vi "ecg_ncs_v1d.vi"() -> ()   [LabVIEW 2016]
uses:
  <instrlib>/niUSRP/niUSRP Timestamp.ctl
  C:/Program Files/National Instruments/LabVIEW 2016/examples/Instrument IO/Serial/support/Serial - Settings.ctl
  <vilib>/Analysis/coordinate.llb/Wrap Angle (array).vi
  <instrlib>/niUSRP/niUSRP Configure Time Start Trigger.vi
  <vilib>/Analysis/3filter.llb/Butterworth Filter (DBL).vi
  <vilib>/Instr/_visa.llb/VISA Configure Serial Port (Instr).vi
  <instrlib>/niUSRP/niUSRP Write Tx Data (2D CDB).vi
  <instrlib>/niUSRP/niUSRP Fetch Rx Data (2D CDB).vi
  <vilib>/measure/NI_MABase.lvlib
  <vilib>/Analysis/NI_AALBase.lvlib
  <vilib>/Analysis/NI_AALPro.lvlib
  <vilib>/Analysis/NI_AAL_Angle.lvlib
panel:
  out "size(s) 5":i32=800
  in  "Stop":bool
  out "size(s) 4":i32=800
  out "x/y":dbl=2000.0
  out "size(s) 3":i32=20000
  out "size(s) 2":i32=10
  out "Poor Sensor Quality: \nSensor off":bool=TRUE
  out "Poor Sensor Quality: \nSensor on":bool
  out "Heart Rate 2":u16[](array[numeric])=[71]
  out "Stop Loop":bool
  out "Loop index":i32=135
  out "size(s)":i32=384
  in  "Read Count":u32=800
  out "return count":u32=800
  out "Serial Settings:Number of Bytes at Serial Port":u32=8
  in  "Serial Settings":T1={"baud rate"=57600, "data bits"=8, "parity"=enum."None", "stop bits"=10, "flow control"=0} {"flow control" items=["None"=0, "XON/XOFF"=1, "RTS/CTS"=2, "DTR/DSR"=4]; "stop bits" items=["1.0"=10, "1.5"=15, "2.0"=20]; "data bits" min=5 max=8 step=1; "baud rate" items=["75"=75, "110"=110, "134"=134, "150"=150, "300"=300, "600"=600, "1200"=1200, "1800"=1800, "2400"=2400, "4800"=4800, "7200"=7200, "9600"=9600, "14400"=14400, "19200"=19200, "28800"=28800, "38400"=38400, "56000"=56000, "57600"=57600, "115200"=115200, "128000"=128000, "230400"=230400]}
  in  "VISA resource name":refnum<visa-resource-name>="bmd101"
  in  "?":enum32{"ECG", "Heart Rate"}(tab)
  out "?":i16(graph)=77
  out "?":u8[](graph)=[71]
  in  "File Name":string="Test"
  in  "order1":i32=5
  in  "Path":path=path "D:/Research/SummerFall17Spring18/CnC/NCS/EcgNcsCorrelation"
  in  "Low-Pass Freq":dbl=200.0 format="%#_13g"
  in  "Sampling Rate":i32=500
  out "Gain":dbl=-15.0
  out "Bandwidth":dbl=56000000.0
  out "Coerced Carrier Frequency":dbl=2000000000.0 format="%#.17g"
  out "Coerced Tx IQ rate":dbl=1000000.0
  out "Coerced Rx IQ rate":dbl=1000000.0
  out "error IO":errorcluster={"status"=FALSE, "code"=-1074118647, "source"=""}
  in  "Rx Number of Samples":i32=20000
  in  "Tab Control 2":enum32{"NI-294x/295x", "NI-2900/2901"}(tab)=enum."NI-2900/2901"
  in  "channel 0 carrier\n frequency [Hz]":dbl=2000000000.0 format="%#_6p"
  in  "Rx carrier frequency [Hz]":dbl=2000000000.0 format="%#_6p"
  in  "Tx carrier frequency [Hz]":dbl=1000000000.0 format="%#_6p"
  in  "Start Trigger Time":T2={"whole seconds"=1, "fractional seconds"=0.0}
  out "Tx Active Antenna":string="TX1"
  in  "Tab Control":T3(tab)
  out "NCS tag Amp":dbl[](graph)=[0.011680657018198379]
  out "NCS tag Phase":dbl[](graph)=[-1.312166394909216]
  out "Tag Amp":dbl[](graph)
  out "Tag Phase":dbl[](graph)
  out "Tx Waveform Graph":waveform(dbl)[](graph)
  in  "Channel 0\nTone Amplitude":dbl=0.707 step=0.05 format="%#.6g"
  in  "Channel 0 \nTone Frequency":dbl=5000.0 format="%#_6p"
  in  "Waveform Size":dbl=20000.0
  in  "Rx Active Antenna":string="RX2"
  in  "Device Name":refnum<k15>="MyB200"
  in  "Tx Gain":dbl=28.0 format="%#_6f"
  in  "Tx IQ Rate":dbl=1000000.0 format="%#_6p"
  in  "Rx Gain":dbl=32.0 format="%#_6f"
  in  "Rx IQ Rate":dbl=1000000.0 format="%#_6p"
  # "Rx Settings"
  # "Tx Settings"
  # "Note that on the NI-2900 and NI-2901, both Rx channels share an LO and both Tx channels share an LO. However, on the NI-294x/295x devices, Rx and Tx of channel 0 share an LO and Rx and Tx of channel 1 share an LO."
  # "This Tx graph should always have end and start tied up since this is being sent in a loop continuously. Otherwise phase jumps will be noticed."
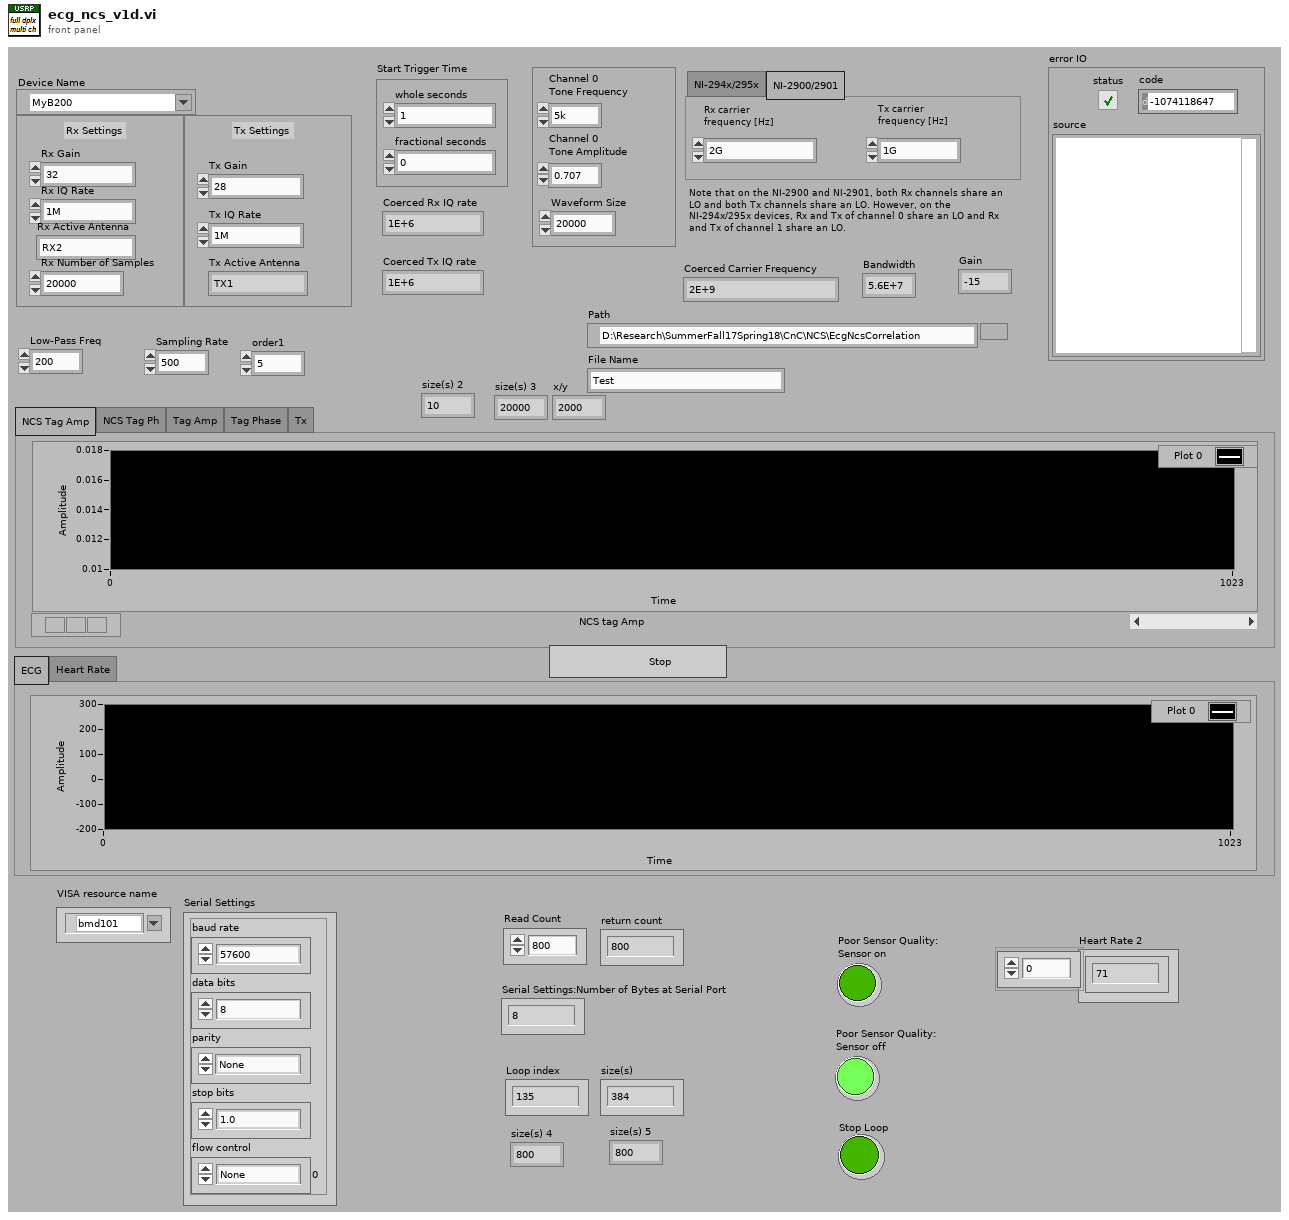
[diagram p1: front panel]
types:
  T1 = typedef "Serial - Settings.ctl" = cluster{"baud rate":u32, "data bits":u16, "parity":enum16{"None", "Odd", "Even", "Mark", "Space"}, "stop bits":u16, "flow control":u16}
  T2 = typedef "niUSRP Timestamp.ctl" = cluster{"whole seconds":u64, "fractional seconds":dbl}
  T3 = enum32{"NCS Tag Amp", "NCS Tag Ph", "Tag Amp", "Tag Phase", "Tx"}
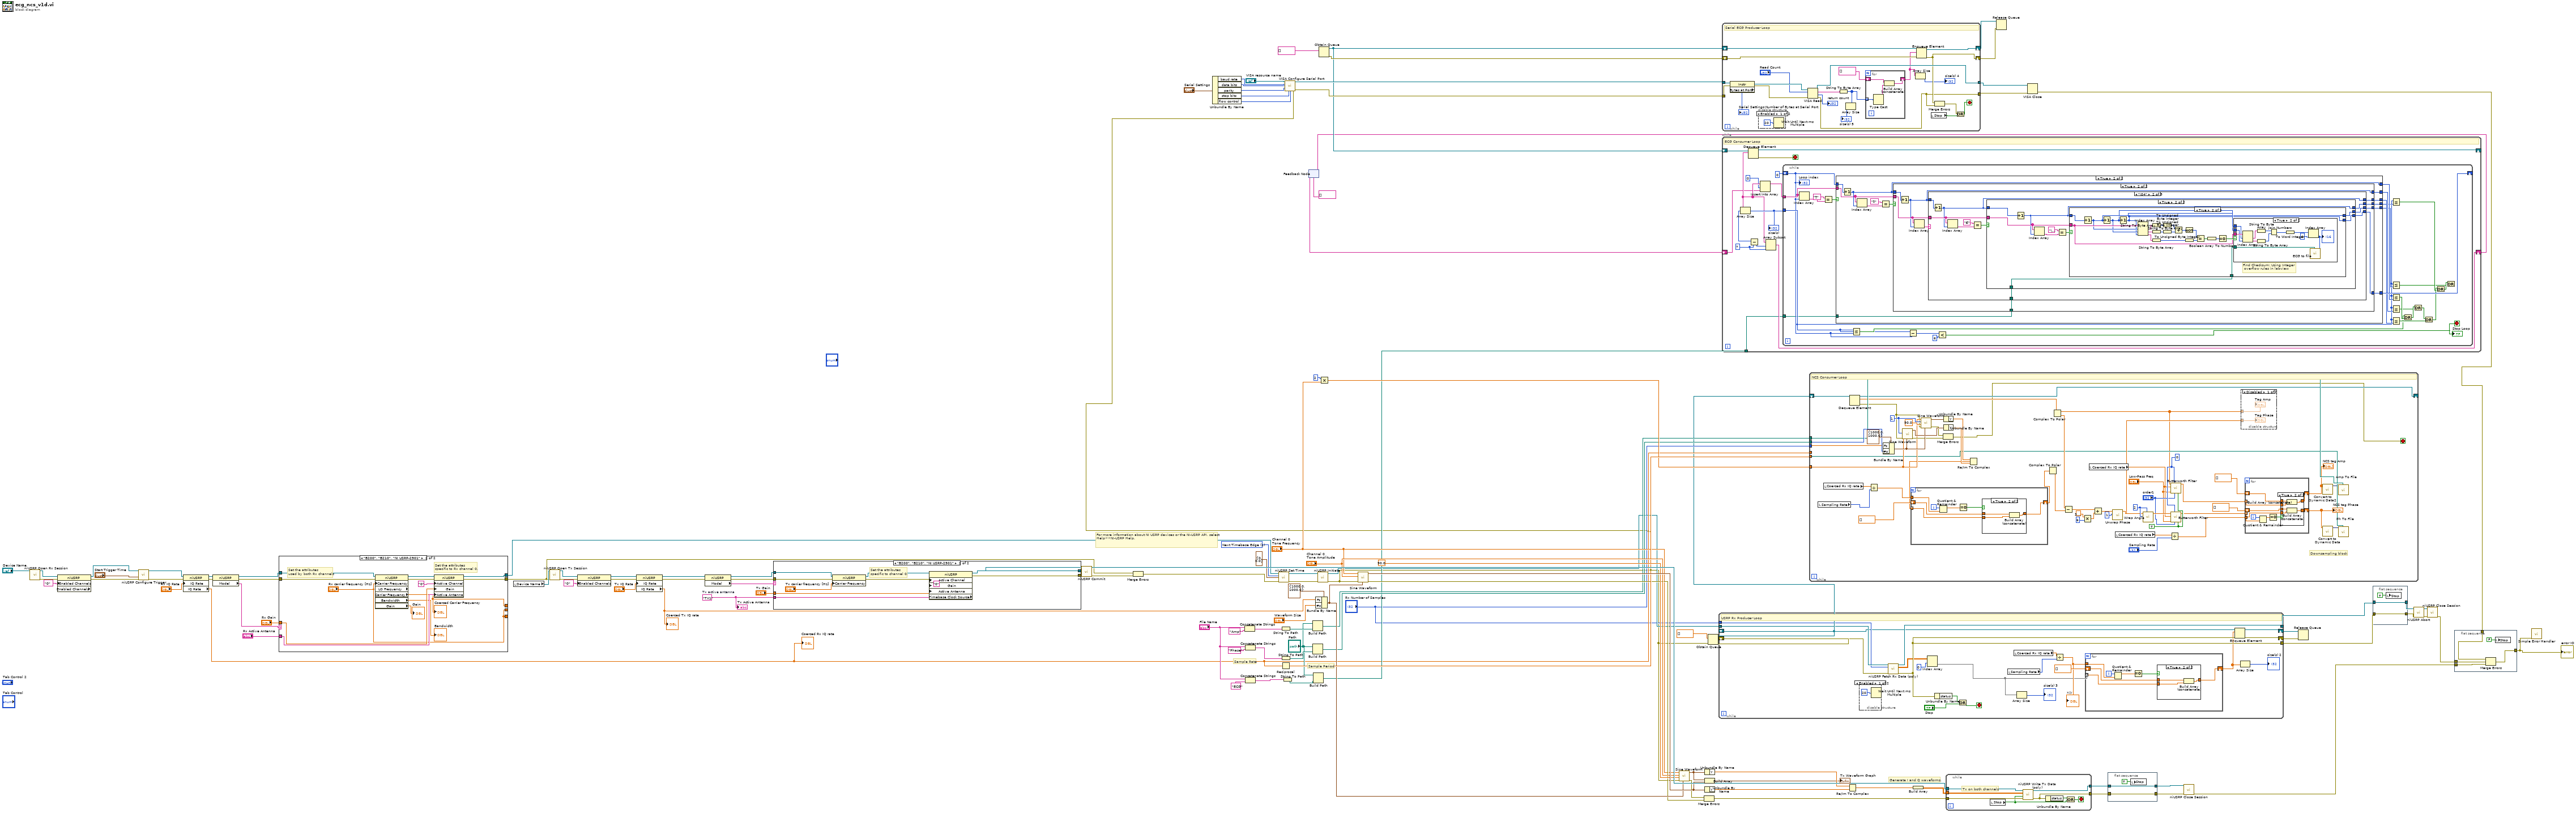
[diagram p0: block diagram]
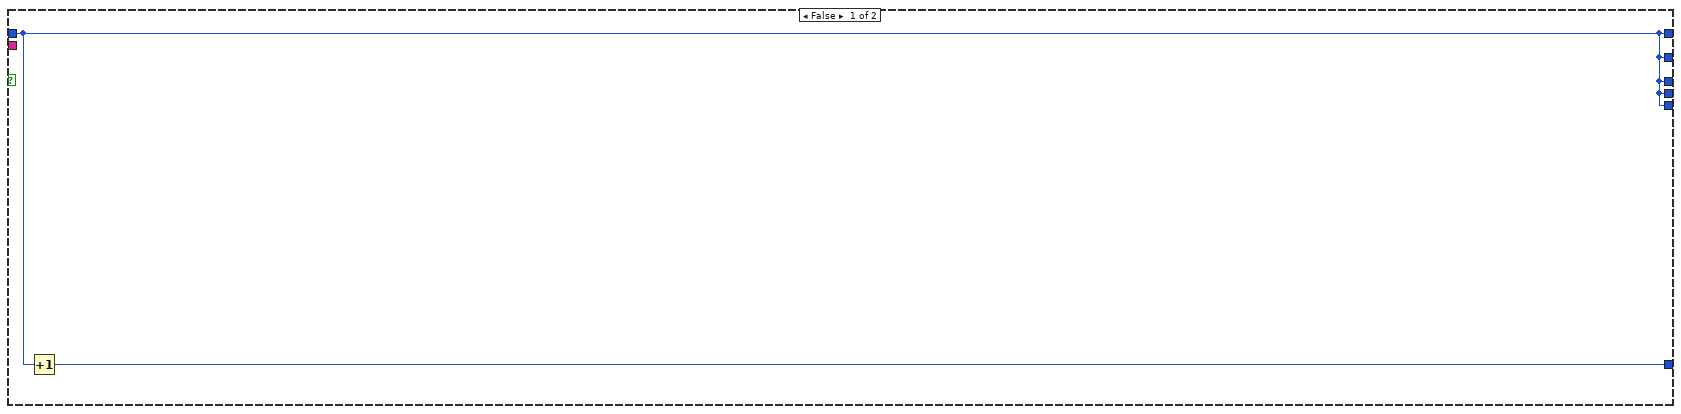
[diagram p4: hidden frame]
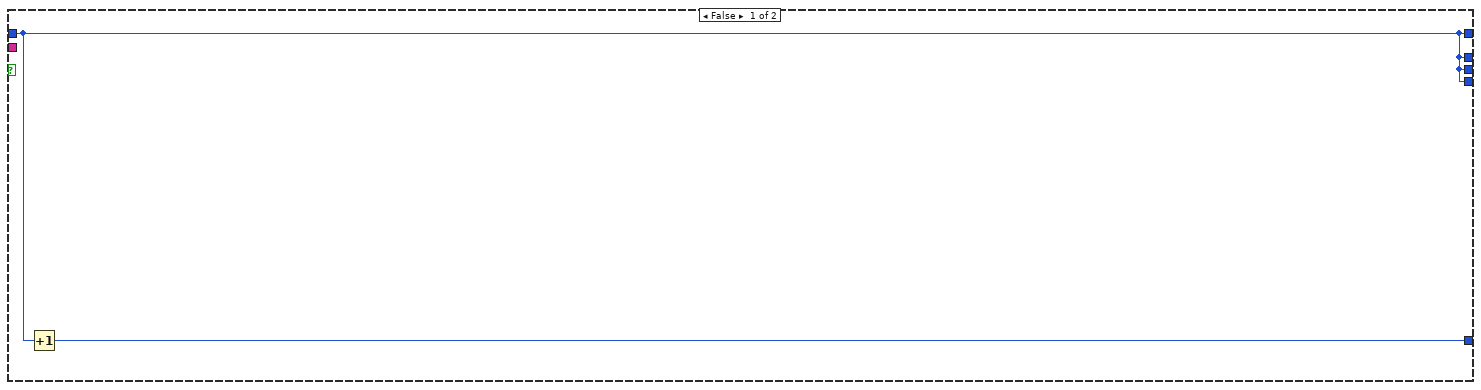
[diagram p5: hidden frame]
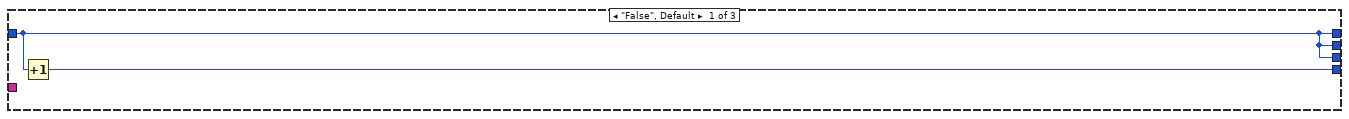
[diagram p6: hidden frame]
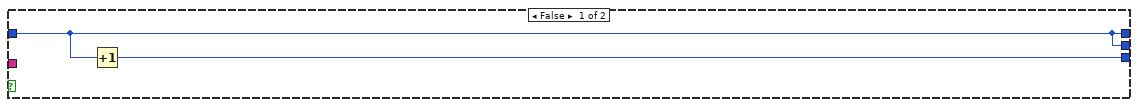
[diagram p7: hidden frame]
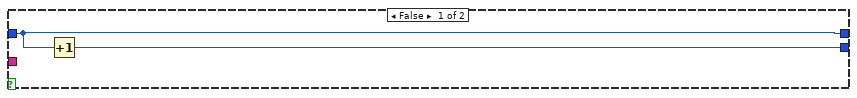
[diagram p8: hidden frame]
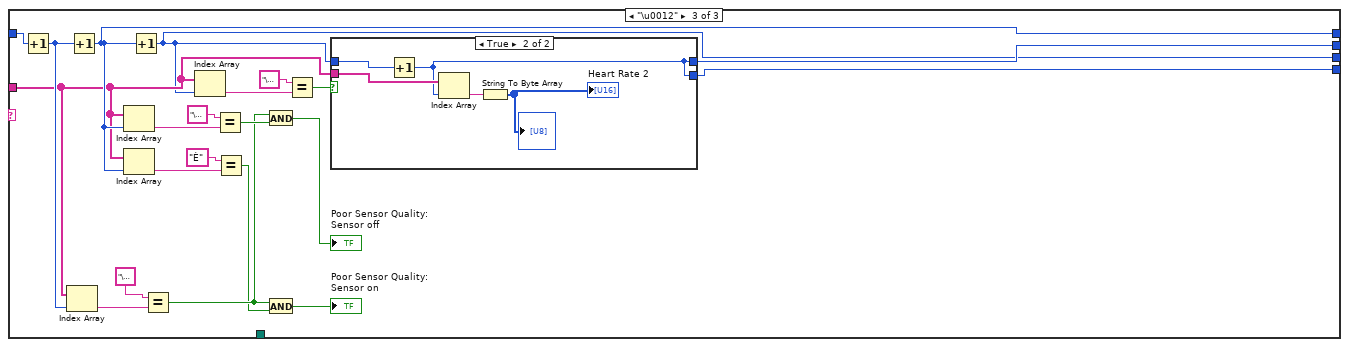
[diagram p10: hidden frame]
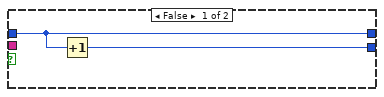
[diagram p11: hidden frame]
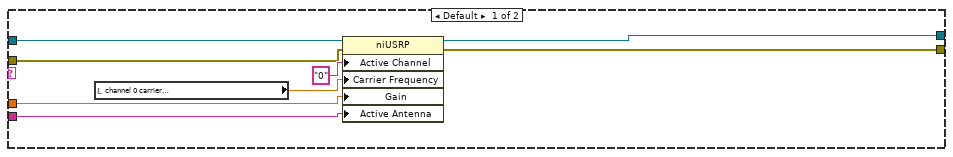
[diagram p13: hidden frame]
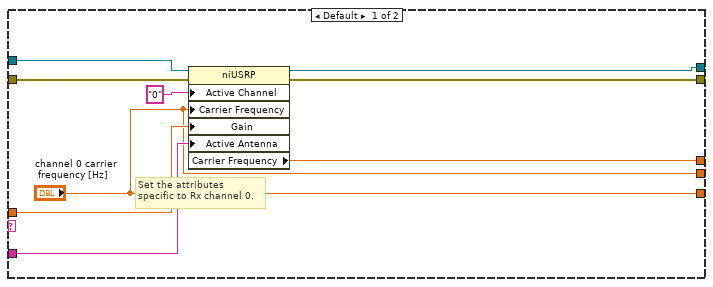
[diagram p14: hidden frame]
diagram:
  w92 = 1 items=["Now", "Next Timebase Edge"] ("apply timestamp")
  w61 = "TX1"  # Tx active antenna
  # "Sample Rate"
  # "Sample Period"
  # "For more information about NI USRP devices or the NI-USRP API, select Help>>NI-USRP Help."
  # "Generate I and Q waveforms."
  n1 = call <instrlib>:"niUSRP Open Rx Session.vi"("device names"="Device Name") -> ("session handle out"=w91:refnum<k15>, "error out"=w90:errorcluster)  [unwired: 13 in]
  n2 = property class="niUSRP" props=["Enabled Channels", "Enabled Channels"](reference=w91, error in=w90, "Enabled Channels"="0" ("Configuration:Enabled Channels")) -> (reference out=w89:refnum<k15>, error out=w88:errorcluster)  [unwired: 1 out]
  n3 = call-poly <instrlib>:"niUSRP Configure Trigger.vi"("session handle"=w89, "start trigger time"="Start Trigger Time", "error in (no error)"=w88) -> ("session handle out"=w85:refnum<k15>, "error out"=w84:errorcluster)  [unwired: 11 in]
  n4 = property class="niUSRP"(reference=w85, error in=w84, "IQ Rate"="Rx IQ Rate") -> (reference out=w81:refnum<k15>, error out=w82:errorcluster, "IQ Rate"=w13:dbl)
  "Coerced Rx IQ rate" <- w13
  n5 = property class="niUSRP"(reference=w81, error in=w82) -> (reference out=w76:refnum<k15>, error out=w77:errorcluster, "Model"=w78:string)
  n6 = case shown="\"B200\", \"B210\", \"NI USRP-2901\"" w78 {
    tunnel: w77 -> [w126 w136]
    tunnel: w76 -> [w125 w137]
    tunnel: [w122 w133] -> w80
    tunnel: [w121 w132] -> w79
    tunnel: "Rx Gain" -> [w124 w139]
    tunnel: "Rx Active Antenna" -> [w123 w138]
    tunnel: [w119 w128] -> _
    tunnel: ["channel 0 carrier\n frequency [Hz]" "Rx carrier frequency [Hz]"] -> _
    tunnel: ["channel 0 carrier\n frequency [Hz]" "Rx carrier frequency [Hz]"] -> _
    frame Default {
      # "Set the attributes \nspecific to Rx channel 0."
      n7 = property class="niUSRP"(reference=w125, error in=w126, "Active Channel"="0", "Carrier Frequency"="channel 0 carrier\n frequency [Hz]", "Gain"=w124, "Active Antenna"=w123) -> (reference out=w122:refnum<k15>, error out=w121:errorcluster, "Carrier Frequency"=w119:dbl)
    }
    frame "B200", "B210", "NI USRP-2901" {
      # "Set the attributes \nused by both Rx channels"
      # "Set the attributes \nspecific to Rx channel 0."
      n8 = property class="niUSRP" props=["Carrier Frequency", "LO Frequency", "Carrier Frequency", "Bandwidth", "Gain"](reference=w137, error in=w136, "Carrier Frequency"="Rx carrier frequency [Hz]") -> (reference out=w135:refnum<k15>, error out=w134:errorcluster, "Carrier Frequency"=w128:dbl, "Bandwidth"=→"Bandwidth":dbl, "Gain"=→"Gain":dbl)  [unwired: 1 out]
      "Coerced Carrier Frequency" <- w128
      n9 = property class="niUSRP"(reference=w135, error in=w134, "Active Channel"="0", "Gain"=w139, "Active Antenna"=w138) -> (reference out=w133:refnum<k15>, error out=w132:errorcluster)
    }
  }
  n10 = local read "Device Name"() -> (w113:refnum<k15>)
  n11 = call <instrlib>:"niUSRP Open Tx Session.vi"("device names"=w113, "error in (no error)"=w79) -> ("session handle out"=w87:refnum<k15>, "error out"=w86:errorcluster)  [unwired: 12 in]
  n12 = property class="niUSRP"(reference=w87, error in=w86, "Enabled Channels"="0" ("Configuration:Enabled Channels")) -> (reference out=w73:refnum<k15>, error out=w72:errorcluster)
  n13 = property class="niUSRP"(reference=w73, error in=w72, "IQ Rate"="Tx IQ Rate") -> (reference out=w67:refnum<k15>, error out=w68:errorcluster, "IQ Rate"=w65:dbl)
  "Coerced Tx IQ rate" <- w65
  n14 = property class="niUSRP"(reference=w67, error in=w68) -> (reference out=w69:refnum<k15>, error out=w70:errorcluster, "Model"=w66:string)
  n15 = case shown="\"B200\", \"B210\", \"NI USRP-2901\"" w66 {
    tunnel: "Tx Gain" -> [w148 w158]
    tunnel: w61 -> [w146 w156]
    tunnel: [w142 w150] -> w63
    tunnel: [w141 w149] -> w64
    tunnel: w70 -> [w145 w152]
    tunnel: w69 -> [w144 w155]
    frame Default {
      n16 = local read "channel 0 carrier\n frequency [Hz]"() -> (w143:dbl)
      n17 = property class="niUSRP"(reference=w144, error in=w145, "Active Channel"="0", "Carrier Frequency"=w143, "Gain"=w148, "Active Antenna"=w146) -> (reference out=w142:refnum<k15>, error out=w141:errorcluster)
    }
    frame "B200", "B210", "NI USRP-2901" {
      # "Set the attributes \nspecific to channel 0."
      n18 = property class="niUSRP"(reference=w155, error in=w152, "Carrier Frequency"="Tx carrier frequency [Hz]") -> (reference out=w154:refnum<k15>, error out=w153:errorcluster)
      n19 = property class="niUSRP" props=["Active Channel", "Gain", "Active Antenna", "Timebase Clock Source"](reference=w154, error in=w153, "Active Channel"="0", "Gain"=w158, "Active Antenna"=w156) -> (reference out=w150:refnum<k15>, error out=w149:errorcluster)  [unwired: 1 out]
    }
  }
  n20 = call <instrlib>:"niUSRP Commit.vi"("session handle"=w63, "error in (no error)"=w64) -> ("session handle out"=w115:refnum<k15>, "error out"=w116:errorcluster)  [unwired: 12 in]
  n21 = Merge Errors(w79, w116) -> (w94:errorcluster)
  n22 = Unbundle By Name("Serial Settings") -> ("baud rate"=w38:u32, "data bits"=w37:u16, "parity"=w36:enum16{"None", "Odd", "Even", "Mark", "Space"}, "stop bits"=w35:u16, "flow control"=w34:u16)
  n23 = Concatenate Strings("File Name", "Amp") -> (w46:string)
  n24 = Concatenate Strings("File Name", "Phase") -> (w43:string)
  n25 = Concatenate Strings("File Name", "ECG") -> (w17:string)
  n26 = call <instrlib>:"niUSRP Set Time.vi"("session handle"=w80, "apply timestamp"=w92, "timestamp"=T2 {"whole seconds"=0, "fractional seconds"=0.0}, "error in (no error)"=w94) -> ("session handle out"=w96:refnum<k15>, "error out"=w95:errorcluster)  [unwired: 10 in]
  n27 = String To Path(string=w46) -> (path=w45:path)
  n28 = String To Path(string=w43) -> (path=w42:path)
  n29 = Reciprocal(x=w13) -> (1/x=w99:dbl)
  n30 = String To Path(string=w17) -> (path=w16:path)
  n31 = feedback #1(string[] []) -> (w22:string[])
  n32 = Build Path(base path="Path", name or relative path=w45) -> (appended path=w48:path)
  n33 = Build Path(base path="Path", name or relative path=w42) -> (appended path=w41:path)
  n34 = Build Path(base path="Path", name or relative path=w16) -> (appended path=w19:path)
  n35 = Bundle By Name(cluster=cluster{"Fs":dbl, "#s":dbl} {"Fs"=1000.0, "#s"=1000.0} ("sampling info"), "Fs"=w65, "#s"="Waveform Size") -> (w98:cluster{"Fs":dbl, "#s":dbl})
  n36 = call <instrlib>:"niUSRP Initiate.vi"("session handle"=w96, "error in (no error)"=w95) -> ("session handle out"=w12:refnum<k15>, "error out"=w8:errorcluster)  [unwired: 12 in]
  n37 = call-poly "VISA Configure Serial Port"("VISA resource name"="VISA resource name", "baud rate (9600)"=w38, "data bits (8)"=w37, "parity (0:none)"=w36, "error in (no error)"=w8, "stop bits (10: 1 bit)"=w35, "flow control (0:none)"=w34) -> ("VISA resource name out"=w30:refnum<visa-resource-name>, "error out"=w29:errorcluster)  [unwired: 3 in, 4 out]
  n38 = Obtain Queue(element data type=string[] []) -> (queue out=w24:refnum<queue>, error out=w26:errorcluster)  [unwired: 4 in, 1 out]
  n39 = Multiply(x=2, y="Channel 0 \nTone Frequency") -> (x*y=w49:dbl)
  n40 = call <vilib>:"Sine Waveform.vi"("sampling info"=w98, "error in (no error)"=w8, "amplitude"="Channel 0\nTone Amplitude", "frequency"="Channel 0 \nTone Frequency") -> ("error out"=w60:errorcluster, "signal out"=w108:waveform(dbl))  [unwired: 6 in]
  n41 = call <vilib>:"Sine Waveform.vi"("sampling info"=w98, "error in (no error)"=w8, "phase"=90.0, "amplitude"="Channel 0\nTone Amplitude", "frequency"="Channel 0 \nTone Frequency") -> ("error out"=w59:errorcluster, "signal out"=w107:waveform(dbl))  [unwired: 5 in]
  n42 = Merge Errors(w59, w60) -> (w58:errorcluster)
  n43 = Unbundle By Name(w107) -> ("Y"=w106:dbl[])
  n44 = Build Array(w107, w108) -> (→"Tx Waveform Graph":waveform(dbl)[])
  n45 = Unbundle By Name(w108) -> ("Y"=w105:dbl[])
  n46 = Obtain Queue(element data type=dbl[] [], error in (no error)=w8) -> (queue out=w3:refnum<queue>, error out=w6:errorcluster)  [unwired: 3 in, 1 out]
  n47 = while {
    tunnel: w12 -> [w179]
    tunnel: [w178] -> w11
    tunnel: "Rx Number of Samples" -> [w177]
    tunnel: [w173] -> w2
    shift-right: [w175] -> w5
    shift-left: w3 -> [w176]
    shift-right: [w174] -> w4
    shift-left: w6 -> [w168]
    stop <- w164 stop-if-true
    # "USRP Rx Producer Loop"
    n48 = disable-structure shown="Enabled" {
      frame Enabled {
        n49 = Wait Until Next ms Multiple(millisecond multiple=u32 20 ("milliseconds to wait")) -> ()  [unwired: 1 out]
      }
      frame Disabled {
      }
    }
    n50 = call-poly <instrlib>:"niUSRP Fetch Rx Data (poly).vi"("session handle"=w179, "number of samples"=w177, "error in (no error)"=w168) -> ("session handle out"=w178:refnum<k15>, "data"=w171:cdb[][], "error out"=w173:errorcluster)  [unwired: 9 in, 1 out]
    n51 = Index Array(array=w171, index (row)=0 ("y")) -> (element=w159:cdb[])  [unwired: 1 in]
    n52 = Unbundle By Name(w173) -> ("status"=w165:bool)
    n53 = Or(x=w165, y="Stop") -> (x .or. y?=w164:bool)
    n54 = local read "Sampling Rate"() -> (w163:i32)
    n55 = local read "Coerced Rx IQ rate"() -> (w167:dbl)
    n56 = Array Size(array=w159) -> (size(s)=→"size(s) 3":i32)
    n57 = Divide(x=w167, y=w163) -> (x/y=w169:dbl)
    "x/y" <- w169
    n58 = for {
      tunnel: w159 -> [w186] mode=indexing
      shift-right: [w184] -> w162
      shift-left: dbl[] [] -> [w185]
      tunnel: w169 -> [w180]
      i -> [w183]
      n59 = Quotient & Remainder(x=w183, y=w180) -> (x-y*floor(x/y)=w181:dbl)  [unwired: 1 out]
      n60 = Equal To 0?(x=w181) -> (x = 0?=w182:bool)
      n61 = case shown="True" w182 {
        tunnel: w186 -> [_ w190]
        tunnel: w185 -> [w187 w189]
        tunnel: [w187 w188] -> w184
        frame False {
        }
        frame True {
          n62 = Build Array (concatenate)(w189, w190) -> (w188:cdb[])
        }
      }
    }
    n63 = Enqueue Element(queue=w176, element=w162, error in (no error)=w173) -> (queue out=w175:refnum<queue>, error out=w174:errorcluster)  [unwired: 1 in, 1 out]
    n64 = Array Size(array=w162) -> (size(s)=→"size(s) 2":i32)
  }
  n65 = while {
    shift-right: [w202] -> _
    shift-left: w24 -> [w203]
    shift-right: [w195] -> w23
    shift-left: w22 -> [w193]
    tunnel: w19 -> [w192]
    stop <- w201 stop-if-true
    w198 = 7
    # "ECG Consumer Loop"
    n66 = Dequeue Element(queue=w203) -> (queue out=w202:refnum<queue>, element=w196:string[], error out=w201:errorcluster)  [unwired: 2 in, 1 out]
    n67 = Array Size(array=w196) -> (size(s)=w200:i32)
    "size(s)" <- w200
    n68 = Subtract(x=w200, y=w198) -> (x-y=w199:i32)
    n69 = Insert Into Array(array=w196, index=0, new element=w193) -> (w197:string[])
    n70 = Array Subset(array=w196, index=w199, length=w198) -> (w195:string[])
    n71 = while {
      tunnel: w197 -> [w226]
      shift-right: [w230] -> _
      shift-left: 0 -> [w209]
      tunnel: w200 -> [w210]
      tunnel: w192 -> [w205]
      stop <- w206 stop-if-true
      n72 = Index Array(array=w226, index=w209) -> (element=w229:string)
      n73 = Equal?(x="ª", y=w229) -> (x = y?=w227:bool)
      n74 = case shown="True" w227 {
        tunnel: w209 -> [w231 w242]
        tunnel: [w232 w240] -> w230
        tunnel: w226 -> [_ w234]
        tunnel: [w231 w239] -> w225
        tunnel: [w231 w238] -> w223
        tunnel: [w231 w237] -> w220
        tunnel: [w231 w236] -> w217
        tunnel: [w231 w235] -> w214
        tunnel: w205 -> [_ w233]
        frame False {
          n75 = Increment(x=w231) -> (x+1=w232:i32)
        }
        frame True {
          n76 = Increment(x=w242) -> (x+1=w239:i32)
          n77 = Index Array(array=w234, index=w239) -> (element=w244:string)
          n78 = Equal?(x="ª", y=w244) -> (x = y?=w241:bool)
          n79 = case shown="True" w241 {
            tunnel: w239 -> [w245 w249]
            tunnel: [w246 w255] -> w240
            tunnel: w234 -> [_ w254]
            tunnel: [w245 w250] -> w238
            tunnel: [w245 w253] -> w237
            tunnel: [w245 w252] -> w236
            tunnel: [w245 w251] -> w235
            tunnel: w233 -> [_ w247]
            frame False {
              n80 = Increment(x=w245) -> (x+1=w246:i32)
            }
            frame True {
              n81 = Increment(x=w249) -> (x+1=w250:i32)
              n82 = Index Array(array=w254, index=w250) -> (element=w248:string)
              n83 = case shown="\"\\04\"" w248 {
                tunnel: w250 -> [w256 w264 w332]
                tunnel: [w257 w263 w314] -> w255
                tunnel: w254 -> [_ w262 w316]
                tunnel: [w256 w261 w318] -> w253
                tunnel: [w256 w260 w315] -> w252
                tunnel: [w256 w259 w313] -> w251
                tunnel: w247 -> [_ w258 _]
                frame "False", Default {
                  n84 = Increment(x=w256) -> (x+1=w257:i32)
                }
                frame "\u0004" {
                  n85 = Increment(x=w264) -> (x+1=w261:i32)
                  n86 = Index Array(array=w262, index=w261) -> (element=w265:string)
                  n87 = Equal?(x="€", y=w265) -> (x = y?=w266:bool)
                  n88 = case shown="True" w266 {
                    tunnel: w261 -> [w268 w275]
                    tunnel: [w269 w274] -> w263
                    tunnel: w262 -> [_ w273]
                    tunnel: [w268 w272] -> w260
                    tunnel: [w268 w271] -> w259
                    tunnel: w258 -> [_ w270]
                    frame False {
                      n89 = Increment(x=w268) -> (x+1=w269:i32)
                    }
                    frame True {
                      n90 = Increment(x=w275) -> (x+1=w272:i32)
                      n91 = Index Array(array=w273, index=w272) -> (element=w276:string)
                      n92 = Equal?(x="\u0002", y=w276) -> (x = y?=w277:bool)
                      n93 = case shown="True" w277 {
                        tunnel: w272 -> [w279 w285]
                        tunnel: [w280 w282] -> w274
                        tunnel: w273 -> [_ w286]
                        tunnel: [w279 w282] -> w271
                        tunnel: w270 -> [_ w281]
                        frame False {
                          n94 = Increment(x=w279) -> (x+1=w280:i32)
                        }
                        frame True {
                          # "Find Checksum: Using Integer\n overflow rules in labview"
                          n95 = Increment(x=w285) -> (x+1=w284:i32)
                          n96 = Increment(x=w284) -> (x+1=w283:i32)
                          n97 = Increment(x=w283) -> (x+1=w282:i32)
                          n98 = Index Array(array=w286, index #1=w284, index #2=w283, index #3=w282) -> (element #1=w300:string, element #2=w299:string, element #3=w293:string)
                          n99 = String To Byte Array(string=w300) -> (unsigned byte array=w298:u8[])
                          n100 = String To Byte Array(string=w299) -> (unsigned byte array=w297:u8[])
                          n101 = String To Byte Array(string=w293) -> (unsigned byte array=w292:u8[])
                          n102 = To Unsigned Byte Integer(number=w298) -> (unsigned 8bit integer=w296:u8[])
                          n103 = To Unsigned Byte Integer(number=w297) -> (unsigned 8bit integer=w295:u8[])
                          n104 = Add(x=w296, y=w295) -> (x+y=w294:u8[])
                          n105 = Not(x=w294) -> (.not. x?=w291:u8[])
                          n106 = To Unsigned Byte Integer(number=w292) -> (unsigned 8bit integer=w290:u8[])
                          n107 = Equal?(x=w291, y=w290) -> (x = y?=w289:bool[])
                          n108 = Boolean Array To Number(Boolean array=w289) -> (number=w288:u32)
                          n109 = Equal To 0?(x=w288) -> (x = 0?=w287:bool)
                          n110 = case shown="True" w287 {
                            tunnel: w286 -> [_ w312]
                            tunnel: w284 -> [_ w306]
                            tunnel: w283 -> [_ w305]
                            tunnel: w281 -> [_ w301]
                            frame False {
                            }
                            frame True {
                              n111 = Index Array(array=w312, index #1=w306, index #2=w305) -> (element #1=w311:string, element #2=w310:string)
                              n112 = String To Byte Array(string=w311) -> (unsigned byte array=w309:u8[])
                              n113 = String To Byte Array(string=w310) -> (unsigned byte array=w308:u8[])
                              n114 = Join Numbers(hi=w309, lo=w308) -> ((hi.lo)=w307:u16[])
                              n115 = To Word Integer(number=w307) -> (16bit integer=w304:i16[])
                              n116 = Index Array(array=w304, index=0) -> (element=w302:i16)
                              "?" <- w302
                              n117 = call "ECG to file"("Signals"=w302, "Filename"=w301) -> ()  [unwired: 15 in, 3 out]
                            }
                          }
                        }
                      }
                    }
                  }
                }
                frame "\u0012" {
                  n118 = Increment(x=w332) -> (x+1=w328:i32)
                  n119 = Index Array(array=w316, index=w328) -> (element=w331:string)
                  n120 = Increment(x=w328) -> (x+1=w318:i32)
                  n121 = Index Array(array=w316, index=w318) -> (element=w329:string)
                  n122 = Index Array(array=w316, index=w318) -> (element=w326:string)
                  n123 = Increment(x=w318) -> (x+1=w313:i32)
                  n124 = Equal?(x="\u0002", y=w331) -> (x = y?=w323:bool)
                  n125 = Index Array(array=w316, index=w313) -> (element=w319:string)
                  n126 = Equal?(x="\u0000", y=w329) -> (x = y?=w325:bool)
                  n127 = Equal?(x="È", y=w326) -> (x = y?=w322:bool)
                  n128 = And(x=w323, y=w325) -> (x .and. y?=→"Poor Sensor Quality: \nSensor off":bool)
                  n129 = And(x=w323, y=w322) -> (x .and. y?=→"Poor Sensor Quality: \nSensor on":bool)
                  n130 = Equal?(x="\u0003", y=w319) -> (x = y?=w317:bool)
                  n131 = case shown="True" w317 {
                    tunnel: w313 -> [w334 w340]
                    tunnel: w316 -> [_ w339]
                    tunnel: [w334 w338] -> w315
                    tunnel: [w335 w338] -> w314
                    frame False {
                      n132 = Increment(x=w334) -> (x+1=w335:i32)
                    }
                    frame True {
                      n133 = Increment(x=w340) -> (x+1=w338:i32)
                      n134 = Index Array(array=w339, index=w338) -> (element=w337:string)
                      n135 = String To Byte Array(string=w337) -> (unsigned byte array=→"Heart Rate 2" →"?":u8[])
                    }
                  }
                }
              }
            }
          }
        }
      }
      n136 = Less Or Equal?(x=w210, y=w209) -> (x <= y?=w211:bool)
      n137 = Subtract(x=w210, y=w209) -> (x-y=w208:i32)
      n138 = Less?(x=w208, y=6) -> (x < y?=w206:bool)
      "Stop Loop" <- w206
      n139 = Less Or Equal?(x=w210, y=w217) -> (x <= y?=w215:bool)
      n140 = Less Or Equal?(x=w210, y=w214) -> (x <= y?=w212:bool)
      n141 = Less Or Equal?(x=w210, y=w225) -> (x <= y?=w224:bool)
      n142 = Less Or Equal?(x=w210, y=w223) -> (x <= y?=w221:bool)
      n143 = Less Or Equal?(x=w210, y=w220) -> (x <= y?=w218:bool)
      n144 = Or(x=w211, y=w224) -> (x .or. y?=w222:bool)
      n145 = Or(x=w222, y=w221) -> (x .or. y?=w219:bool)
      n146 = Or(x=w219, y=w218) -> (x .or. y?=w216:bool)
      n147 = Or(x=w216, y=w215) -> (x .or. y?=w213:bool)
      n148 = Or(x=w213, y=w212) -> ()  [unwired: 1 out]
      "Loop index" <- w209
    }
  }
  n149 = feedback-in #1(w23) -> ()
  n150 = while {
    tunnel: w29 -> [w351]
    tunnel: [w355] -> w32
    shift-right: [w356] -> w28
    shift-left: w26 -> [w359]
    shift-right: [w357] -> w25
    shift-left: w24 -> [w358]
    tunnel: w30 -> [w353]
    tunnel: [w360] -> w31
    stop <- w362 stop-if-true
    # "Serial ECG Producer Loop"
    n151 = property class="Instr"(reference=w353, error in=w351) -> (reference out=w352:refnum<visa-resource-name>, error out=w350:errorcluster, "Bytes at Port"=→"Serial Settings:Number of Bytes at Serial Port":u32)
    n152 = disable-structure shown="Enabled" {
      frame Enabled {
        n153 = Wait Until Next ms Multiple(millisecond multiple=u32 20 ("milliseconds to wait")) -> ()  [unwired: 1 out]
      }
      frame Disabled {
      }
    }
    n154 = VISA Read(VISA resource name=w352, byte count="Read Count", error in (no error)=w350) -> (VISA resource name out=w360:refnum<visa-resource-name>, read buffer=w341:string, return count=→"return count":u32, error out=w355:errorcluster)
    n155 = String To Byte Array(string=w341) -> (unsigned byte array=w343:u8[])
    n156 = Array Size(array=w343) -> (size(s)=→"size(s) 5":i32)
    n157 = for {
      tunnel: w343 -> [w367] mode=indexing
      shift-right: [w365] -> w344
      shift-left: string[] [] -> [w366]
      n158 = Type Cast(x=w367) -> (*(type *) &x=w364:string)  [unwired: 1 in]
      n159 = Build Array (concatenate)(w366, w364) -> (w365:string[])
    }
    n160 = Array Size(array=w344) -> (size(s)=→"size(s) 4":i32)
    n161 = Enqueue Element(queue=w358, element=w344, error in (no error)=w359) -> (queue out=w357:refnum<queue>, error out=w356:errorcluster)  [unwired: 1 in, 1 out]
    n162 = local read "Stop"() -> (w348:bool)
    n163 = Merge Errors(w356, w355) -> (w354:errorcluster)
    n164 = Or(x=w354, y=w348) -> (x .or. y?=w362:bool)
  }
  n165 = while {
    tunnel: w99 -> [_]
    tunnel: "Rx Number of Samples" -> [w419]
    tunnel: w13 -> [w411]
    tunnel: w49 -> [w412]
    tunnel: w48 -> [w406]
    tunnel: w41 -> [w386]
    shift-right: [w374] -> _
    shift-left: w3 -> [w375]
    stop <- w369 stop-if-true
    w397 = 2 ("y")
    w391 = TRUE
    w393 = 0
    w417 = 1
    # "Downsampling block"
    # "NCS Consumer Loop"
    n166 = local read "Sampling Rate"() -> (w379:i32)
    n167 = local read "Coerced Rx IQ rate"() -> (w380:dbl)
    n168 = Dequeue Element(queue=w375) -> (queue out=w374:refnum<queue>, element=w373:dbl[], error out=w368:errorcluster)  [unwired: 2 in, 1 out]
    n169 = Divide(x=w380, y=w379) -> (x/y=w378:dbl)
    n170 = Bundle By Name(cluster=cluster{"Fs":dbl, "#s":dbl} {"Fs"=1000.0, "#s"=1000.0} ("sampling info"), "Fs"=w411, "#s"=w419) -> (w416:cluster{"Fs":dbl, "#s":dbl})
    n171 = call <vilib>:"Sine Waveform.vi"("sampling info"=w416, "error in (no error)"=w368, "amplitude"=w417, "frequency"=w412) -> ("error out"=w415:errorcluster, "signal out"=w420:waveform(dbl))  [unwired: 6 in]
    n172 = call <vilib>:"Sine Waveform.vi"("sampling info"=w416, "error in (no error)"=w368, "phase"=90.0, "amplitude"=w417, "frequency"=w412) -> ("error out"=w414:errorcluster, "signal out"=w413:waveform(dbl))  [unwired: 5 in]
    n173 = Merge Errors(w414, w415) -> (w369:errorcluster)
    n174 = Unbundle By Name(w413) -> ("Y"=w405:dbl[])
    n175 = Unbundle By Name(w420) -> ("Y"=w404:dbl[])
    n176 = Re/Im To Complex(1:w404, 2:w405) -> (0:w376:cdb[])
    n177 = for {
      tunnel: w376 -> [w428] mode=indexing
      shift-right: [w422] -> w372
      shift-left: dbl[] [] -> [w427]
      tunnel: w378 -> [w423]
      i -> [w426]
      n178 = Quotient & Remainder(x=w426, y=w423) -> (x-y*floor(x/y)=w424:dbl)  [unwired: 1 out]
      n179 = Equal To 0?(x=w424) -> (x = 0?=w425:bool)
      n180 = case shown="True" w425 {
        tunnel: w428 -> [_ w432]
        tunnel: w427 -> [w429 w431]
        tunnel: [w429 w430] -> w422
        frame False {
        }
        frame True {
          n181 = Build Array (concatenate)(w431, w432) -> (w430:cdb[])
        }
      }
    }
    n182 = Complex To Polar(r * e^(i*theta)=w372) -> (theta=w371:dbl[])  [unwired: 1 out]
    n183 = Complex To Polar(r * e^(i*theta)=w373) -> (r=w370:dbl[], theta=w395:dbl[])
    n184 = Subtract(x=w395, y=w371) -> (x-y=w399:dbl[])
    n185 = Multiply(x=3.141592653589793, y=6) -> (x*y=w400:dbl)
    n186 = local read "Coerced Rx IQ rate"() -> (w381:dbl)
    n187 = Add(x=w399, y=w400) -> (x+y=w398:dbl[])
    n188 = call <vilib>:"Unwrap Phase.vi"("phase unit"=1 ("y"), "Phase"=w398) -> ("Unwrapped Phase"=w396:dbl[])  [unwired: 8 in, 1 out]
    n189 = local read "Coerced Rx IQ rate"() -> (w409:dbl)
    n190 = call-poly <vilib>:"Wrap Angle.vi"("angle units"=w397, "angle range"=w397, "Angle In"=w396) -> ("Angle Out"=w394:dbl[])  [unwired: 7 in, 1 out]
    n191 = Divide(x=w409, y="Sampling Rate") -> (x/y=w407:dbl)
    n192 = call-poly <vilib>:"Butterworth Filter.vi"("init/cont (init:F)"=w391, "order"="order1", "filter type"=w393, "low cutoff freq: fl"="Low-Pass Freq", "sampling freq: fs"=w381, "X"=w370) -> ("Filtered X"=w382:dbl[])  [unwired: 2 in, 1 out]
    n193 = call-poly <vilib>:"Butterworth Filter.vi"("init/cont (init:F)"=w391, "order"="order1", "filter type"=w393, "low cutoff freq: fl"="Low-Pass Freq", "sampling freq: fs"=w381, "X"=w394) -> ("Filtered X"=w389:dbl[])  [unwired: 2 in, 1 out]
    n194 = disable-structure shown="Disabled" {
      disable-tunnel: w394 -> [w434 _]
      disable-tunnel: w370 -> [w433 _]
      frame Disabled {
        "Tag Amp" <- w433
        "Tag Phase" <- w434
      }
      frame Enabled {
      }
    }
    n195 = for {
      tunnel: w382 -> [w444] mode=indexing
      shift-right: [w442] -> w384
      shift-left: dbl[] [] -> [w443]
      tunnel: w407 -> [w438]
      shift-right: [w436] -> w387
      shift-left: dbl[] [] -> [w437]
      tunnel: w389 -> [w435] mode=indexing
      i -> [w441]
      n196 = Quotient & Remainder(x=w441, y=w438) -> (x-y*floor(x/y)=w439:dbl)  [unwired: 1 out]
      n197 = Equal To 0?(x=w439) -> (x = 0?=w440:bool)
      n198 = case shown="True" w440 {
        tunnel: w444 -> [_ w452]
        tunnel: w443 -> [w446 w451]
        tunnel: [w446 w450] -> w442
        tunnel: w437 -> [w445 w449]
        tunnel: [w445 w448] -> w436
        tunnel: w435 -> [_ w447]
        frame False {
        }
        frame True {
          n199 = Build Array (concatenate)(w451, w452) -> (w450:dbl[])
          n200 = Build Array (concatenate)(w449, w447) -> (w448:dbl[])
        }
      }
    }
    "NCS tag Amp" <- w384
    "NCS tag Phase" <- w387
    n201 = call "Convert to Dynamic Data2"("Array"=w384) -> ("Dynamic Data Type"=w383:dynamicdata)  [unwired: 3 in]
    n202 = call "Convert to Dynamic Data"("Array"=w387) -> ("Dynamic Data Type"=w388:dynamicdata)  [unwired: 3 in]
    n203 = call "Amp To File"("Signals"=w383, "Filename"=w406) -> ()  [unwired: 15 in, 3 out]
    n204 = call "Ph To File"("Signals"=w388, "Filename"=w386) -> ()  [unwired: 15 in, 3 out]
  }
  n205 = Re/Im To Complex(1:w105, 2:w106) -> (0:w101:cdb[])
  n206 = Build Array(w101) -> (w100:cdb[][])
  n207 = while {
    tunnel: w115 -> [w460]
    tunnel: w58 -> [w459]
    tunnel: [w457] -> w57
    tunnel: [w455] -> w54
    tunnel: w100 -> [w454]
    stop <- w456 stop-if-true
    # "Tx on both channels"
    n208 = local read "Stop"() -> (w453:bool)
    n209 = call-poly <instrlib>:"niUSRP Write Tx Data (poly).vi"("session handle"=w460, "data"=w454, "end of data?"=w453, "error in (no error)"=w459) -> ("session handle out"=w455:refnum<k15>, "error out"=w457:errorcluster)  [unwired: 10 in]
    n210 = Unbundle By Name(w457) -> ("status"=w458:bool)
    n211 = Compound Arithmetic op=OR(w458, w453) -> (w456:bool)
  }
  n212 = Release Queue(queue=w25, error in (no error)=w28) -> ()  [unwired: 1 in, 3 out]
  n213 = VISA Close(VISA resource name=w31, error in (no error)=w32) -> (error out=w20:errorcluster)
  n214 = flat-sequence {
    tunnel: [w462] -> w56
    tunnel: w57 -> [w462]
    tunnel: [w461] -> w55
    tunnel: w54 -> [w461]
    frame #0 {
      n215 = local write "Stop"(TRUE ("STOP")) -> ()
    }
  }
  n216 = call <instrlib>:"niUSRP Close Session.vi"("session handle"=w55, "error in (no error)"=w56) -> ("error out"=w53:errorcluster)  [unwired: 13 in]
  n217 = Release Queue(queue=w5, error in (no error)=w4) -> ()  [unwired: 1 in, 3 out]
  n218 = flat-sequence {
    tunnel: w11 -> [w465]
    tunnel: [w465] -> w10
    tunnel: w2 -> [w464]
    tunnel: [w464] -> w1
    frame #0 {
      n219 = local write "Stop"(TRUE ("STOP")) -> ()
    }
  }
  n220 = call <instrlib>:"niUSRP Abort.vi"("session handle"=w10, "error in (no error)"=w1) -> ("session handle out"=w112:refnum<k15>, "error out"=w111:errorcluster)  [unwired: 12 in]
  n221 = call <instrlib>:"niUSRP Close Session.vi"("session handle"=w112, "error in (no error)"=w111) -> ("error out"=w52:errorcluster)  [unwired: 13 in]
  n222 = flat-sequence {
    tunnel: w53 -> [w470]
    tunnel: [w469] -> w40
    tunnel: w52 -> [w468]
    tunnel: w20 -> [w467]
    frame #0 {
      n223 = Merge Errors(w467, w468, w470) -> (w469:errorcluster)
      n224 = local write "Stop"(FALSE ("STOP")) -> ()
    }
  }
  n225 = call <vilib>:"Simple Error Handler.vi"("error in (no error)"=w40) -> ()  [unwired: 1 in, 8 out]
  "Tx Active Antenna" <- w61
  "error IO" <- w40
